vi "CRYSet Graph Cluster Data.vi"(11 "Graph Number":i32) -> (3 "DataType":string)   [LabVIEW 2013]
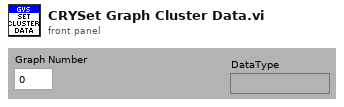
[diagram p1: front panel]
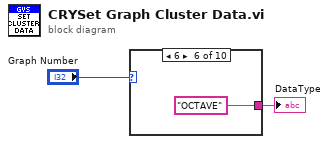
[diagram p0: block diagram]
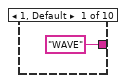
[diagram p2: hidden frame]
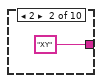
[diagram p3: hidden frame]
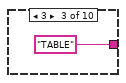
[diagram p4: hidden frame]
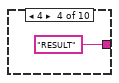
[diagram p5: hidden frame]
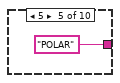
[diagram p6: hidden frame]
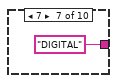
[diagram p7: hidden frame]
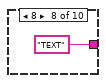
[diagram p8: hidden frame]
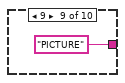
[diagram p9: hidden frame]
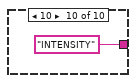
[diagram p10: hidden frame]
diagram:
  n1 = case shown="6" "Graph Number" {
    tunnel: ["WAVE" ("DataType") "XY" ("DataType") "TABLE" ("DataType") "RESULT" ("DataType") "POLAR" ("DataType") "OCTAVE" ("DataType") "DIGITAL" ("DataType") "TEXT" ("DataType") "PICTURE" ("DataType") "INTENSITY" ("DataType")] -> w1
    frame 1, Default {
    }
    frame 2 {
    }
    frame 3 {
    }
    frame 4 {
    }
    frame 5 {
    }
    frame 6 {
    }
    frame 7 {
    }
    frame 8 {
    }
    frame 9 {
    }
    frame 10 {
    }
  }
  "DataType" <- w1
